vi "serial_init_sub.vi"(0 "VISA resource name":refnum<visa-resource-name>="COM7", 1 "baud rate":u32=115200, 2 "data bits":u16=8 min=5 max=8 step=1, 3 "parity":u16(ring) items=["None", "Odd", "Even", "Mark", "Space"], 4 "stop bits":u16(ring)=10 items=["1.0"=10, "1.5"=15, "2.0"=20], 7 "flow control":u16(ring) items=["None"=0, "XON/XOFF"=1, "RTS/CTS"=2, "DTR/DSR"=4]) -> ()   [LabVIEW 2017]
doc: "The Basic Serial Read and Write example performs a Serial Port Read, a Serial Port Write, or a combination of these actions. The user selects the actions (read or write) on the front panel. If both are selected, the VI will write the data first, read data, and then close the VISA session that is opened to the port. This VI will wait until the specified number of bytes is received at the port. Only the number of bytes specified will be read.\n\nINSTRUCTIONS:\n1) Select the serial resource and configuration parameters (baud rate, data bits, parity, stop bits, flow control).\n2) Select the operations to be performed. \n3) Connect the serial port to your device. If no device is available, perform a loopback test by doing one of the following. Short pins 2 and 3 on a RS-232 cable or short pin 4 to pin 8 and pin 5 to pin 9 on a RS-485/422 cable. \n4) Run the VI to see the data read. (The \"read string\" will match the \"string to write\" if a loopback test was performed.)\n\nNote: The parameters set for the serial port must match the parameters of the connected instrument or device. In this example, the bytes to read parameter specifies the number of bytes that the serial port reads. If there were more bytes at the port than the number specified in bytes to read, those bytes would not be read. Also, if you specify to read more bytes than the number of bytes actually read, you might receive a timeout error message.\n\nOn the block diagram, the Configure Serial Port VI sets the configuration parameters. The front panel displays the controls used to configure the basic parameters, such as baud rate, data bits, and parity. Constants configure the other parameters the user probably does not need set. After the VISA Configure Serial Port VI opens the VISA session and configures the port, the VI passes the VISA resource name to other VIs that perform operations on that VISA resource. The VISA Write function sends a command to the serial device and the VISA Read function returns data based on the command. The VISA Close function then closes the reference to the serial device. It is important to close the reference; otherwise communication through with that port through protocols other than VISA might not be possible."
panel:
  out "i":i32
  in  "Success":i32
  out "read string":string
  out "error out":errorcluster
  out "VISA out":refnum<visa-resource-name>="COM7"
  in  "wbc":dbl=1.0
  in  "delay before read (ms)":u32=265
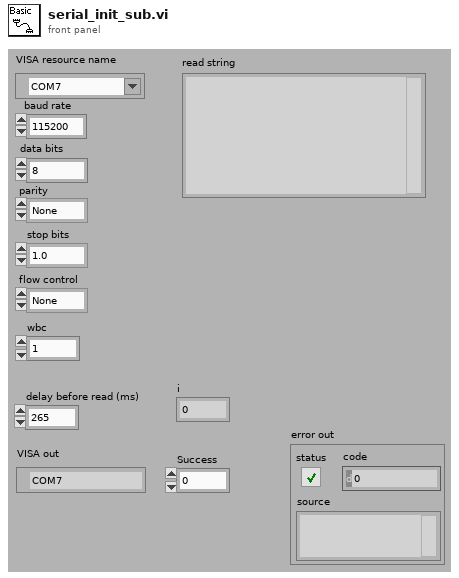
[diagram p1: front panel]
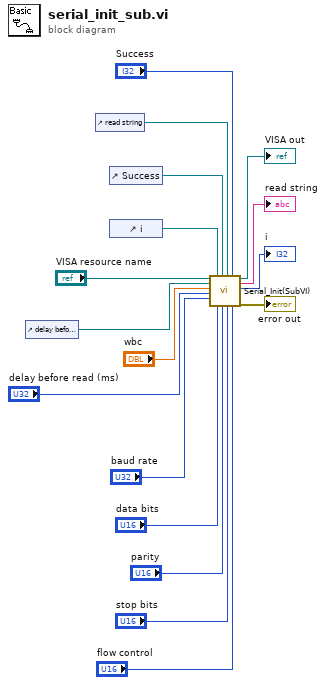
[diagram p0: block diagram]
diagram:
  n1 = control-ref of="delay before read (ms)"() -> (w6:refnum<vi>)
  n2 = control-ref of="read string"() -> (w9:refnum<vi>)
  n3 = control-ref of="Success"() -> (w8:refnum<vi>)
  n4 = control-ref of="i"() -> (w7:refnum<vi>)
  n5 = call "Serial_Init(SubVI).vi"("VISA Refnum in"="VISA resource name", "reference 3"=w6, "wbc"="wbc", "delay before read (ms)"="delay before read (ms)", "baud rate"="baud rate", "reference 4"=w7, "data bits"="data bits", "reference 2"=w8, "parity"="parity", "reference"=w9, "stop bits"="stop bits", "Success"="Success", "flow control"="flow control") -> ("VISA Refnum out"=→"VISA out":refnum<visa-resource-name>, "read string"=→"read string":string, "i"=→"i":i32, "error out"=→"error out":errorcluster)  [unwired: 3 in]
